vi "DrawPhasorPlot.vi"(0 "Intensity":dbl[][](array[numeric]), 1 "G Data":dbl[][](array[numeric]), 2 "S Data":dbl[][](array[numeric]), 3 "Threshold (max)":dbl=0.0035, 4 "Threshold (min)":dbl=0.002, 5 "error in":errorcluster, 6 "G_max":dbl=1.1, 7 "Auto Scale?":bool=TRUE, 8 "G_min":dbl=-0.1, 9 "Phasor Grids":i32, 10 "S_max":dbl=1.1, 11 "Reference":refnum<vi>, 12 "S_min":dbl=-0.1, 13 "Phasor Colormap":T1(ring)=enum."rainbow") -> (14 "Phasor Plot":dbl[][](array[numeric]), 19 "error out":errorcluster)   [LabVIEW 2018]
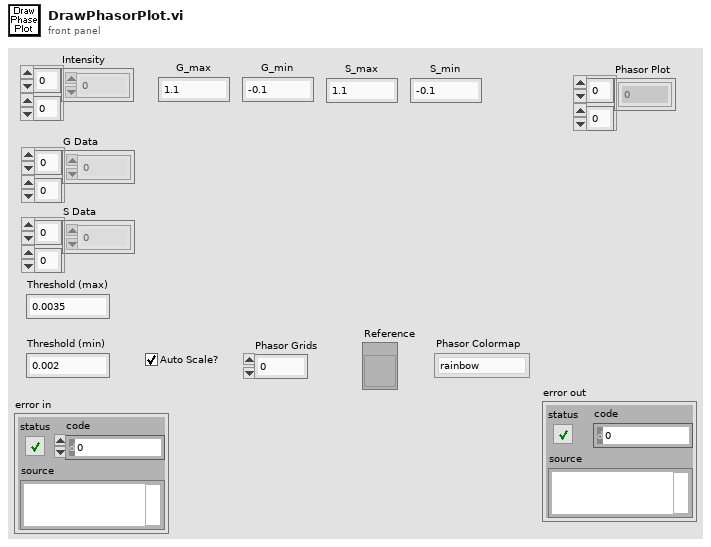
[diagram p1: front panel]
types:
  T1 = enum16{"fire", "rainbow", "gray", "inverse gray", "ice", "original"}
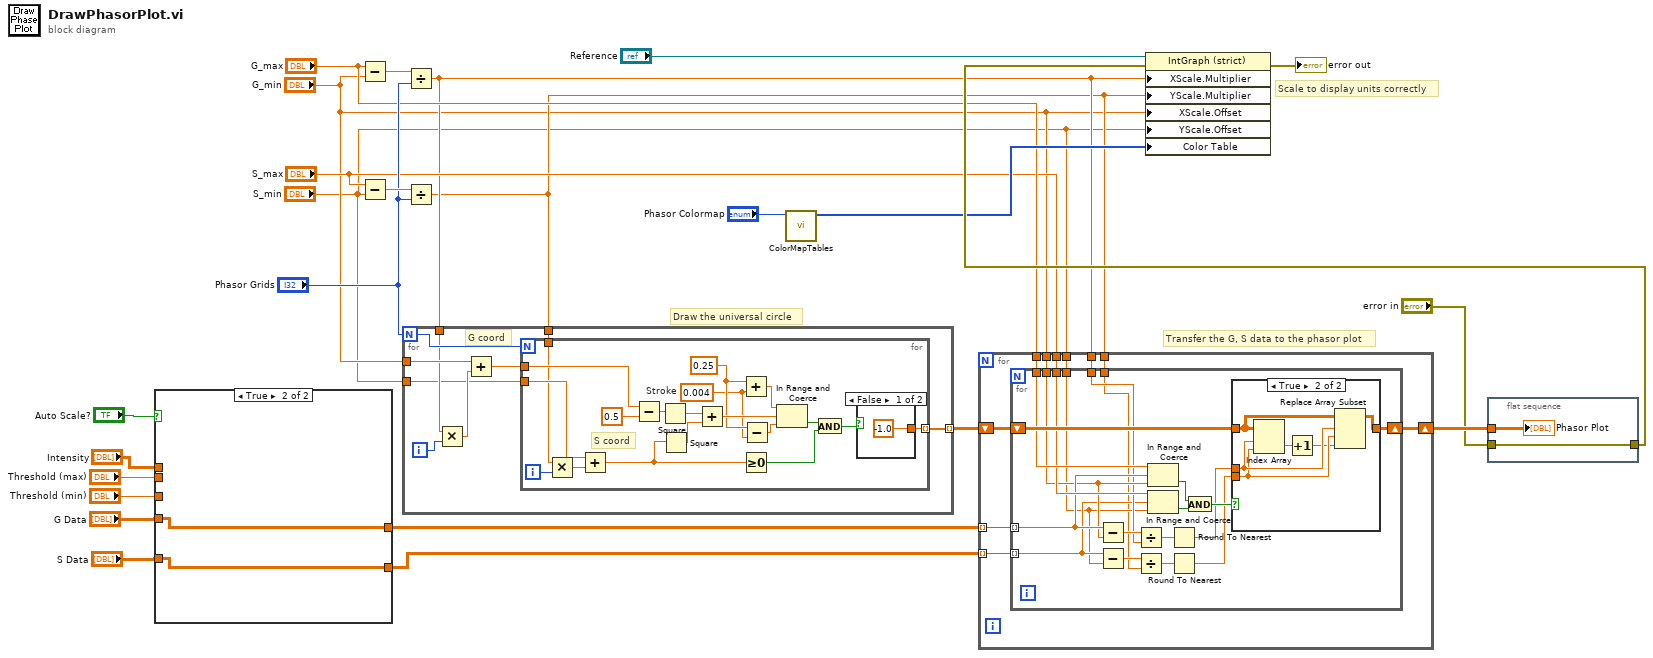
[diagram p0: block diagram]
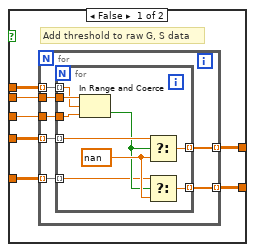
[diagram p2: hidden frame]
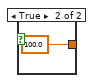
[diagram p4: hidden frame]
diagram:
  # "Scale to display units correctly"
  # "Transfer the G, S data to the phasor plot"
  # "Draw the universal circle"
  n1 = case shown="True" "Auto Scale?" {
    tunnel: "Intensity" -> [w32 _]
    tunnel: "Threshold (max)" -> [w31 _]
    tunnel: "Threshold (min)" -> [w30 _]
    tunnel: "G Data" -> [w29 w50]
    tunnel: "S Data" -> [w28 w49]
    tunnel: [w27 w50] -> w23
    tunnel: [w26 w49] -> w22
    frame False {
      # "Add threshold to raw G, S data"
      n2 = for {
        tunnel: w32 -> [w39] mode=indexing
        tunnel: w31 -> [w38]
        tunnel: [w37] -> w27 mode=indexing
        tunnel: w30 -> [w36]
        tunnel: w29 -> [w35] mode=indexing
        tunnel: w28 -> [w34] mode=indexing
        tunnel: [w33] -> w26 mode=indexing
        n3 = for {
          tunnel: w39 -> [w45] mode=indexing
          tunnel: w38 -> [w47]
          tunnel: [w48] -> w37 mode=indexing
          tunnel: w36 -> [w46]
          tunnel: w35 -> [w44] mode=indexing
          tunnel: w34 -> [w41] mode=indexing
          tunnel: [w40] -> w33 mode=indexing
          w43 = nan ("f")
          n4 = In Range and Coerce(upper limit=w47, x=w45, lower limit=w46) -> (In Range?=w42:bool)  [unwired: 1 out]
          n5 = Select(t=w44, s=w42, f=w43) -> (s? t:f=w48:dbl)
          n6 = Select(t=w41, s=w42, f=w43) -> (s? t:f=w40:dbl)
        }
      }
    }
    frame True {
    }
  }
  n7 = Subtract(x="G_max", y="G_min") -> (x-y=w13:dbl)
  n8 = Subtract(x="S_max", y="S_min") -> (x-y=w12:dbl)
  n9 = Divide(x=w13, y="Phasor Grids") -> (x/y=w4:dbl)
  n10 = Divide(x=w12, y="Phasor Grids") -> (x/y=w3:dbl)
  n11 = for {
    N: "Phasor Grids" -> [w59]
    tunnel: [w58] -> w25 mode=indexing
    tunnel: "G_min" -> [w57]
    tunnel: w4 -> [w54]
    tunnel: "S_min" -> [w52]
    tunnel: w3 -> [w51]
    i -> [w56]
    # "G coord"
    n12 = Multiply(x=w54, y=w56) -> (x*y=w55:dbl)
    n13 = Add(x=w57, y=w55) -> (x+y=w53:dbl)
    n14 = for {
      N: w59 -> [_]
      tunnel: w53 -> [w78]
      tunnel: [w71] -> w58 mode=indexing
      tunnel: w52 -> [w70]
      tunnel: w51 -> [w68]
      i -> [w69]
      w64 = 0.004  # Stroke
      w65 = 0.25 ("x")
      # "S coord"
      n15 = Multiply(x=w68, y=w69) -> (x*y=w67:dbl)
      n16 = Add(x=w70, y=w67) -> (x+y=w63:dbl)
      n17 = Subtract(x=w78, y=0.5) -> (x-y=w77:dbl)
      n18 = Square(x=w77) -> (x^2=w76:dbl)
      n19 = Square(x=w63) -> (x^2=w75:dbl)
      n20 = Add(x=w76, y=w75) -> (x+y=w74:dbl)
      n21 = Add(x=w65, y=w64) -> (x+y=w73:dbl)
      n22 = Greater Or Equal To 0?(x=w63) -> (x >= 0?=w60:bool)
      n23 = Subtract(x=w65, y=w64) -> (x-y=w72:dbl)
      n24 = In Range and Coerce(upper limit=w73, x=w74, lower limit=w72) -> (In Range?=w62:bool)  [unwired: 1 out]
      n25 = And(x=w62, y=w60) -> (x .and. y?=w61:bool)
      n26 = case shown="False" w61 {
        tunnel: [-1.0 ("element") 100.0 ("element")] -> w71
        frame False {
        }
        frame True {
        }
      }
    }
  }
  n27 = call "ColorMapTables.vi"("Map Selector"="Phasor Colormap") -> ("Color Map Array"=w7:u32[])  [unwired: 10 in]
  n28 = for {
    tunnel: w23 -> [w90] mode=indexing
    tunnel: w22 -> [w89] mode=indexing
    shift-right: [w87] -> w24
    shift-left: w25 -> [w88]
    tunnel: "G_max" -> [w86]
    tunnel: "G_min" -> [w85]
    tunnel: "S_max" -> [w84]
    tunnel: "S_min" -> [w83]
    tunnel: w4 -> [w82]
    tunnel: w3 -> [w81]
    n29 = for {
      tunnel: w90 -> [w102] mode=indexing
      tunnel: w89 -> [w96] mode=indexing
      shift-right: [w105] -> w87
      shift-left: w88 -> [w106]
      tunnel: w86 -> [w104]
      tunnel: w85 -> [w101]
      tunnel: w84 -> [w103]
      tunnel: w83 -> [w95]
      tunnel: w82 -> [w99]
      tunnel: w81 -> [w93]
      n30 = Subtract(x=w102, y=w101) -> (x-y=w100:dbl)
      n31 = Subtract(x=w96, y=w95) -> (x-y=w94:dbl)
      n32 = Divide(x=w100, y=w99) -> (x/y=w98:dbl)
      n33 = Divide(x=w94, y=w93) -> (x/y=w92:dbl)
      n34 = In Range and Coerce(upper limit=w104, x=w102, lower limit=w101) -> (In Range?=w109:bool)  [unwired: 1 out]
      n35 = In Range and Coerce(upper limit=w103, x=w96, lower limit=w95) -> (In Range?=w108:bool)  [unwired: 1 out]
      n36 = Round To Nearest(number=w98) -> (nearest integer value=w97:dbl)
      n37 = Round To Nearest(number=w92) -> (nearest integer value=w91:dbl)
      n38 = And(x=w109, y=w108) -> (x .and. y?=w107:bool)
      n39 = case shown="True" w107 {
        tunnel: w106 -> [w110 w115]
        tunnel: w97 -> [_ w114]
        tunnel: w91 -> [_ w113]
        tunnel: [w110 w111] -> w105
        frame False {
        }
        frame True {
          n40 = Index Array(array=w115, index (row)=w114, index (col)=w113) -> (element=w116:dbl)
          n41 = Increment(x=w116) -> (x+1=w112:dbl)
          n42 = Replace Array Subset(array=w115, new element=w112, index (row)=w114, index (col)=w113) -> (w111:dbl[][])
        }
      }
    }
  }
  n43 = property on="Property Node" class="IntGraph (strict)"(reference="Reference", error in=w10, "XScale.Multiplier"=w4, "YScale.Multiplier"=w3, "XScale.Offset"="G_min", "YScale.Offset"="S_min", "Color Table"=w7) -> (error out=→"error out":errorcluster)  [unwired: 1 out]
  n44 = flat-sequence {
    tunnel: w24 -> [w118]
    tunnel: "error in" -> [w117]
    tunnel: [w117] -> w10
    frame #0 {
      "Phasor Plot" <- w118
    }
  }
